vi "Memory.Pointer.Read Bytes.vi"   [LabVIEW 2016, in "LabVIEW Memory Manager.lvlib" / "Memory.Pointer.lvclass"]
uses:
  Memory.Pointer.lvclass
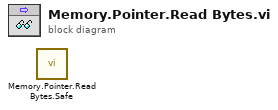
[diagram p0: block diagram]
diagram:
  n1 = call "Memory.Pointer.Read Bytes.Safe.vi"() -> ()  [unwired: 9 in, 3 out]
